vi "Transcriptor LabVIEW to C code Arduino Frontend 2.vi"(11 "vi path":path=path "C:/Users/lubo/Documents/LabView/LabVIEW-Universal-Transcriptor/Test/Examples For Parsing/Example Shift Register Loop 1.vi") -> (3 "transcripted code":string)   [LabVIEW 2014]
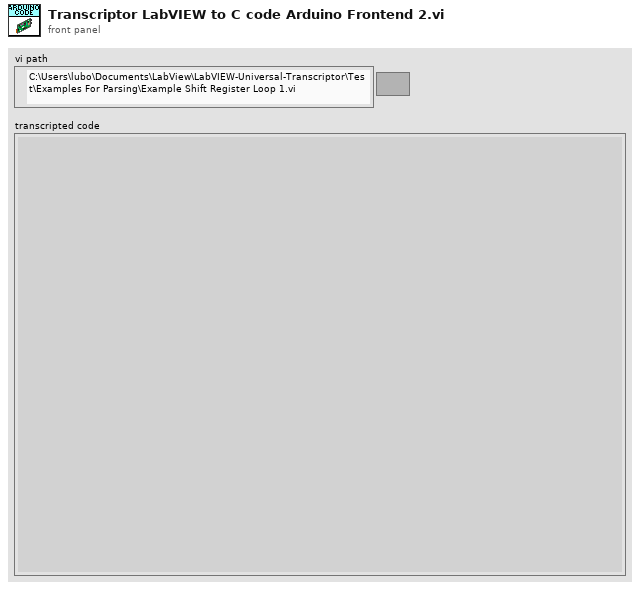
[diagram p1: front panel]
types:
  T1 = typedef "LabVIEW Universal Transcriptor Cluster.ctl" = cluster{"Defines":string[], "Includes":string[], "C code":string, "temp":string[], "temp 2":string[]}
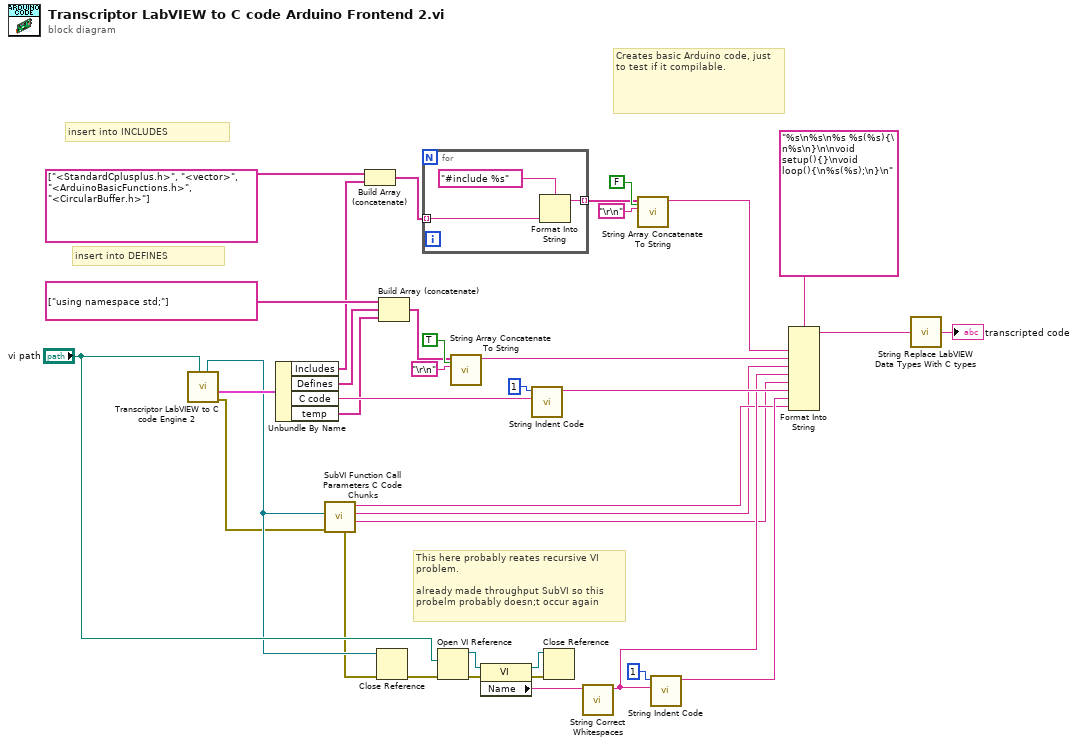
[diagram p0: block diagram]
diagram:
  # "This here probably reates recursive VI problem.\n\nalready made throughput SubVI so this probelm probably doesn;t occur again"
  # "insert into INCLUDES"
  # "insert into DEFINES"
  # "Creates basic Arduino code, just to test if it compilable."
  n1 = call "Transcriptor LabVIEW to C code Engine 2.vi"("VI path"="vi path") -> ("Error Out"=w2:errorcluster, "output cluster"=w37:T1, "VI ref."=w3:refnum<vi>)  [unwired: 6 in, 2 out]
  n2 = Unbundle By Name(w37) -> ("Includes"=w14:string[], "Defines"=w17:string[], "C code"=w25:string, "temp"=w5:string[])
  n3 = call "SubVI Function Call Parameters C Code Chunks.vi"("Error In"=w2, "VI Reference"=w3) -> ("SubVI func. declaration"=w9:string, "return datatype"=w10:string, "SubVI func. call in code"=w11:string, "Error Out"=w1:errorcluster)  [unwired: 4 in, 2 out]
  n4 = Build Array (concatenate)(string[] ["<StandardCplusplus.h>", "<vector>", "<ArduinoBasicFunctions.h>", "<CircularBuffer.h>"], w14) -> (w13:string[])
  n5 = Close Reference(reference=w3, error in (no error)=w1) -> (error out=w4:errorcluster)
  n6 = Build Array (concatenate)(string[] ["using namespace std;"], w17, w5) -> (w16:string[])
  n7 = for {
    tunnel: w13 -> [w39] mode=indexing
    tunnel: [w38] -> w29 mode=indexing
    n8 = Format Into String(format string="#include %s", w39) -> (resulting string=w38:string)  [unwired: 2 in, 1 out]
  }
  n9 = Open VI Reference(vi path="vi path", error in (no error)=w4) -> (vi reference=w7:refnum<vi>, error out=w28:errorcluster)  [unwired: 4 in]
  n10 = call "String Array Concatenate To String.vi"("insert last delimiter?"=TRUE, "Delimiter char"="\r\n", "Array String In"=w16) -> ("String"=w34:string)  [unwired: 8 in]
  n11 = property class="VI"(reference=w7, error in=w28) -> (reference out=w8:refnum<vi>, error out=w26:errorcluster, "Name"=w27:string)
  n12 = call "String Indent Code.vi"("complete code"=w25, "actual nested level"=1) -> ("indented code"=w24:string)  [unwired: 9 in]
  n13 = Close Reference(reference=w8, error in (no error)=w26) -> ()  [unwired: 1 out]
  n14 = call "String Correct Whitespaces.vi"("String in"=w27) -> ("String out"=w21:string)  [unwired: 10 in]
  n15 = call "String Array Concatenate To String.vi"("insert last delimiter?"=FALSE, "Delimiter char"="\r\n", "Array String In"=w29) -> ("String"=w30:string)  [unwired: 8 in]
  n16 = call "String Indent Code.vi"("complete code"=w21, "actual nested level"=1) -> ("indented code"=w20:string)  [unwired: 9 in]
  n17 = Format Into String(format string="%s\n%s\n%s %s(%s){\n%s\n}\n\nvoid setup(){}\nvoid loop(){\n%s(%s);\n}\n", w30, w34, w10, w21, w9, w24, w20, w11) -> (resulting string=w19:string)  [unwired: 2 in, 1 out]
  n18 = call "String Replace LabVIEW Data Types With C types.vi"("C code"=w19) -> ("C code, replaced datatypes"=→"transcripted code":string)
